vi "pp3_updateSideState.vi"(8 "error in (no error)":errorcluster, 9 "log queue in":refnum<queue>, 10 "Daq config In":T1={"Sound AO"="Dev6/ao0", "Shock intesity AO"="Dev6/ao1", "Code_LED DO"="Dev6/port1:2", "Switch DI"="Dev6/port1/line0", "Webcam"="cam9", "Sound AO task"="", "Sound card task"=0, "Shock intensity AO task"="", "Code_LED DO task"="", "Switch DI task"="", "AO <=> Sound card"=FALSE, "Sound card"=0, "sample rate"=100000.0, "Variable shock"=TRUE, "Webcam on"=FALSE, "Waveform memo"={"t0"=timestamp(0 s since 1904-01-01), "dt"=1.0, "Y"=[]}, "First time"=FALSE, "Tone trigger"="", "Master-9 DO"="Dev6/port0/line5:7"} {"sample rate" min=8000.0; "Sound card task" format="%.0x"}, 11 "State In":T4={"Curr  tr"=0, "Curr (ms)"=0, "Cum (ms)"=0, "Run loop diff"=0, "Tone countdown (ms)"=0, "Countdown (ms)"=0, "Curr State"=enum."0 NULL", "Prev State"=enum."1 Habituation", "Rw"=FALSE, "Sw"=FALSE, "Tone\nGate"=FALSE, "Punish"=FALSE, "Current DAQ DO Int"=0, "Current Loaded Trial"={"Trial Type Number"=1, "Trial Type"=enum."GO", "Trial Weight"=100, "Shock (mA)"=0.3, "Duration (ms)"=0.25, "Sound Type"=enum."04 FM Sweep", "Stim P1"=4000.0, "Stim P2"=0.0, "Stim P3"=0.0, "Stim P4"=2000.0, "DAQ Amplitude (V)"=0.25}, "Next Trial (for display purposes)"={"Trial Type Number"=1, "Trial Type"=enum."GO", "Trial Weight"=100, "Shock (mA)"=0.3, "Duration (ms)"=0.25, "Sound Type"=enum."04 FM Sweep", "Stim P1"=4000.0, "Stim P2"=0.0, "Stim P3"=0.0, "Stim P4"=2000.0, "DAQ Amplitude (V)"=0.25}, "Total trials memo"=0, "State start cum memo (ms)"=0, "Last dur jump time memo (ms)"=0, "Last dur shock time memo (ms)"=0, "Tone repeat memo (ms)"=0, "Webcam on"=FALSE, "Webcam recording"=FALSE, "State update flag"=FALSE, "Last loaded shock voltage"=0.0, "Vid upd"=enum."0"} {"Current DAQ DO Int" format="%016b"; "Next Trial (for display purposes)"."DAQ Amplitude (V)" min=0.0 max=5.0 format="%_4g"; "Next Trial (for display purposes)"."Shock (mA)" min=-1.0 max=5.0; "Next Trial (for display purposes)"."Trial Weight" step=1; "Next Trial (for display purposes)"."Duration (ms)" min=0.0 max=1.0; "Next Trial (for display purposes)"."Trial Type Number" min=1 max=256 step=1; "Current Loaded Trial"."DAQ Amplitude (V)" min=0.0 max=5.0 format="%_4g"; "Current Loaded Trial"."Shock (mA)" min=-1.0 max=5.0; "Current Loaded Trial"."Trial Weight" step=1; "Current Loaded Trial"."Duration (ms)" min=0.0 max=1.0; "Current Loaded Trial"."Trial Type Number" min=1 max=256 step=1}) -> (0 "error out":errorcluster, 1 "log queue out":refnum<queue>, 3 "State Out":T4={"Curr  tr"=0, "Curr (ms)"=0, "Cum (ms)"=0, "Run loop diff"=0, "Tone countdown (ms)"=0, "Countdown (ms)"=0, "Curr State"=enum."0 NULL", "Prev State"=enum."1 Habituation", "Rw"=FALSE, "Sw"=FALSE, "Tone\nGate"=FALSE, "Punish"=FALSE, "Current DAQ DO Int"=0, "Current Loaded Trial"={"Trial Type Number"=1, "Trial Type"=enum."GO", "Trial Weight"=100, "Shock (mA)"=0.3, "Duration (ms)"=0.25, "Sound Type"=enum."04 FM Sweep", "Stim P1"=4000.0, "Stim P2"=0.0, "Stim P3"=0.0, "Stim P4"=2000.0, "DAQ Amplitude (V)"=0.25}, "Next Trial (for display purposes)"={"Trial Type Number"=1, "Trial Type"=enum."GO", "Trial Weight"=100, "Shock (mA)"=0.3, "Duration (ms)"=0.25, "Sound Type"=enum."04 FM Sweep", "Stim P1"=4000.0, "Stim P2"=0.0, "Stim P3"=0.0, "Stim P4"=2000.0, "DAQ Amplitude (V)"=0.25}, "Total trials memo"=0, "State start cum memo (ms)"=0, "Last dur jump time memo (ms)"=0, "Last dur shock time memo (ms)"=0, "Tone repeat memo (ms)"=0, "Webcam on"=FALSE, "Webcam recording"=FALSE, "State update flag"=FALSE, "Last loaded shock voltage"=0.0, "Vid upd"=enum."0"} {"Current DAQ DO Int" format="%016b"; "Next Trial (for display purposes)"."DAQ Amplitude (V)" min=0.0 max=5.0 format="%_4g"; "Next Trial (for display purposes)"."Shock (mA)" min=-1.0 max=5.0; "Next Trial (for display purposes)"."Trial Weight" step=1; "Next Trial (for display purposes)"."Duration (ms)" min=0.0 max=1.0; "Next Trial (for display purposes)"."Trial Type Number" min=1 max=256 step=1; "Current Loaded Trial"."DAQ Amplitude (V)" min=0.0 max=5.0 format="%_4g"; "Current Loaded Trial"."Shock (mA)" min=-1.0 max=5.0; "Current Loaded Trial"."Trial Weight" step=1; "Current Loaded Trial"."Duration (ms)" min=0.0 max=1.0; "Current Loaded Trial"."Trial Type Number" min=1 max=256 step=1}, 4 "State timeout":bool, 5 "vid display":bool, 6 "Side change":bool)   [LabVIEW 2013]
uses:
  pp3_CTL_StateInfo.ctl
  pp3_CTL_State.ctl
  pp3_CTL_Trial.ctl
  pp3_CTL_TrialType.ctl
  labolabo2/waveforms/WFTypes.ctl
  pp3_CTL_DaqConfig.ctl
  <vilib>/userdefined/High Color/IMAQdx.ctl
  <vilib>/sound2/lvsound2.llb/Sound Output Task ID.ctl
  <vilib>/DAQmx/read.llb/DAQmx Read (Digital Bool 1Line 1Point).vi
  <vilib>/DAQmx/miscellaneous.llb/DAQmx Fill In Error Info.vi
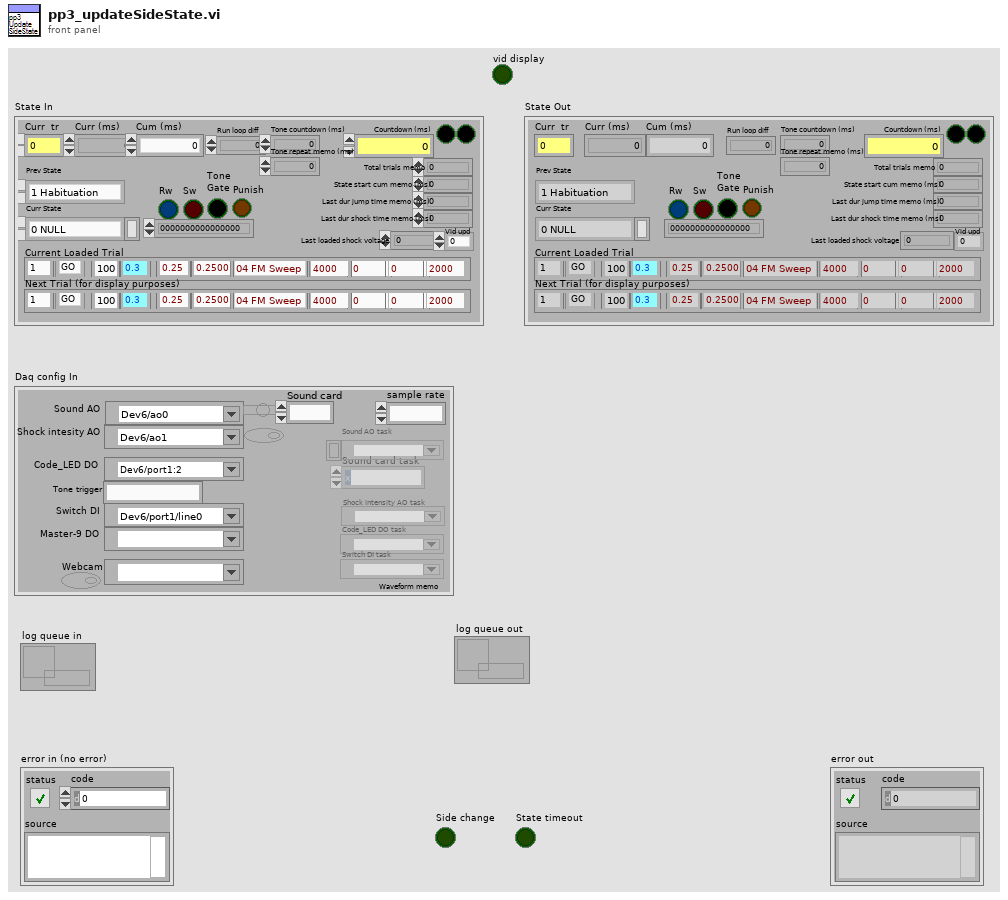
[diagram p1: front panel]
types:
  T1 = typedef "pp3_CTL_DaqConfig.ctl" = cluster{"Sound AO":tag, "Shock intesity AO":tag, "Code_LED DO":tag, "Switch DI":tag, "Webcam":T2, "Sound AO task":refnum<k21>, "Sound card task":T3, "Shock intensity AO task":refnum<k21>, "Code_LED DO task":refnum<k21>, "Switch DI task":refnum<k21>, "AO <=> Sound card":bool, "Sound card":u32, "sample rate":dbl, "Variable shock":bool, "Webcam on":bool, "Waveform memo":waveform(dbl), "First time":bool, "Tone trigger":string, "Master-9 DO":tag}
  T2 = typedef "IMAQdx.ctl" = refnum<k21>
  T3 = typedef "Sound Output Task ID.ctl" = u32
  T4 = typedef "pp3_CTL_StateInfo.ctl" = cluster{"Curr  tr":u16, "Curr (ms)":u32, "Cum (ms)":i64, "Run loop diff":i64, "Tone countdown (ms)":i64, "Countdown (ms)":i64, "Curr State":T5, "Prev State":T5, "Rw":bool, "Sw":bool, "Tone\nGate":bool, "Punish":bool, "Current DAQ DO Int":u16, "Current Loaded Trial":T6, "Next Trial (for display purposes)":T6, "Total trials memo":i64, "State start cum memo (ms)":i64, "Last dur jump time memo (ms)":i64, "Last dur shock time memo (ms)":i64, "Tone repeat memo (ms)":i64, "Webcam on":bool, "Webcam recording":bool, "State update flag":bool, "Last loaded shock voltage":dbl, "Vid upd":enum16{"0", "1", "2", "3", "4", "5", "6", "7", "8", "9"}}
  T5 = typedef "pp3_CTL_State.ctl" = enum8{"0 NULL", "1 Habituation", "2 (Load Trial)", "3 Stay Period", "4 Load Audio/Click Delay", "5 GO Trial", "6 GO Jumped", "7 GO Timeout", "8 NOGO Trial", "9 NOGO Jumped", "10 NOGO Timeout", "11 TEST Trial", "12 TEST Jumped", "13 TEST Timeout", "14 Intertrial Interval", "15 Done"}
  T6 = typedef "pp3_CTL_Trial.ctl" = cluster{"Trial Type Number":i16, "Trial Type":T7, "Trial Weight":u32, "Shock (mA)":dbl, "Duration (ms)":dbl, "Sound Type":T8, "Stim P1":dbl, "Stim P2":dbl, "Stim P3":dbl, "Stim P4":dbl, "DAQ Amplitude (V)":dbl}
  T7 = typedef "pp3_CTL_TrialType.ctl" = enum16{"OFF", "GO", "NOGO", "TEST"}
  T8 = typedef "WFTypes.ctl" = enum16{"00 NULL", "01 DC", "02 Noise", "03 Pure Tone", "04 FM Sweep"}
  T9 = enum16{"0", "1", "2", "3", "4", "5", "6", "7", "8", "9"}
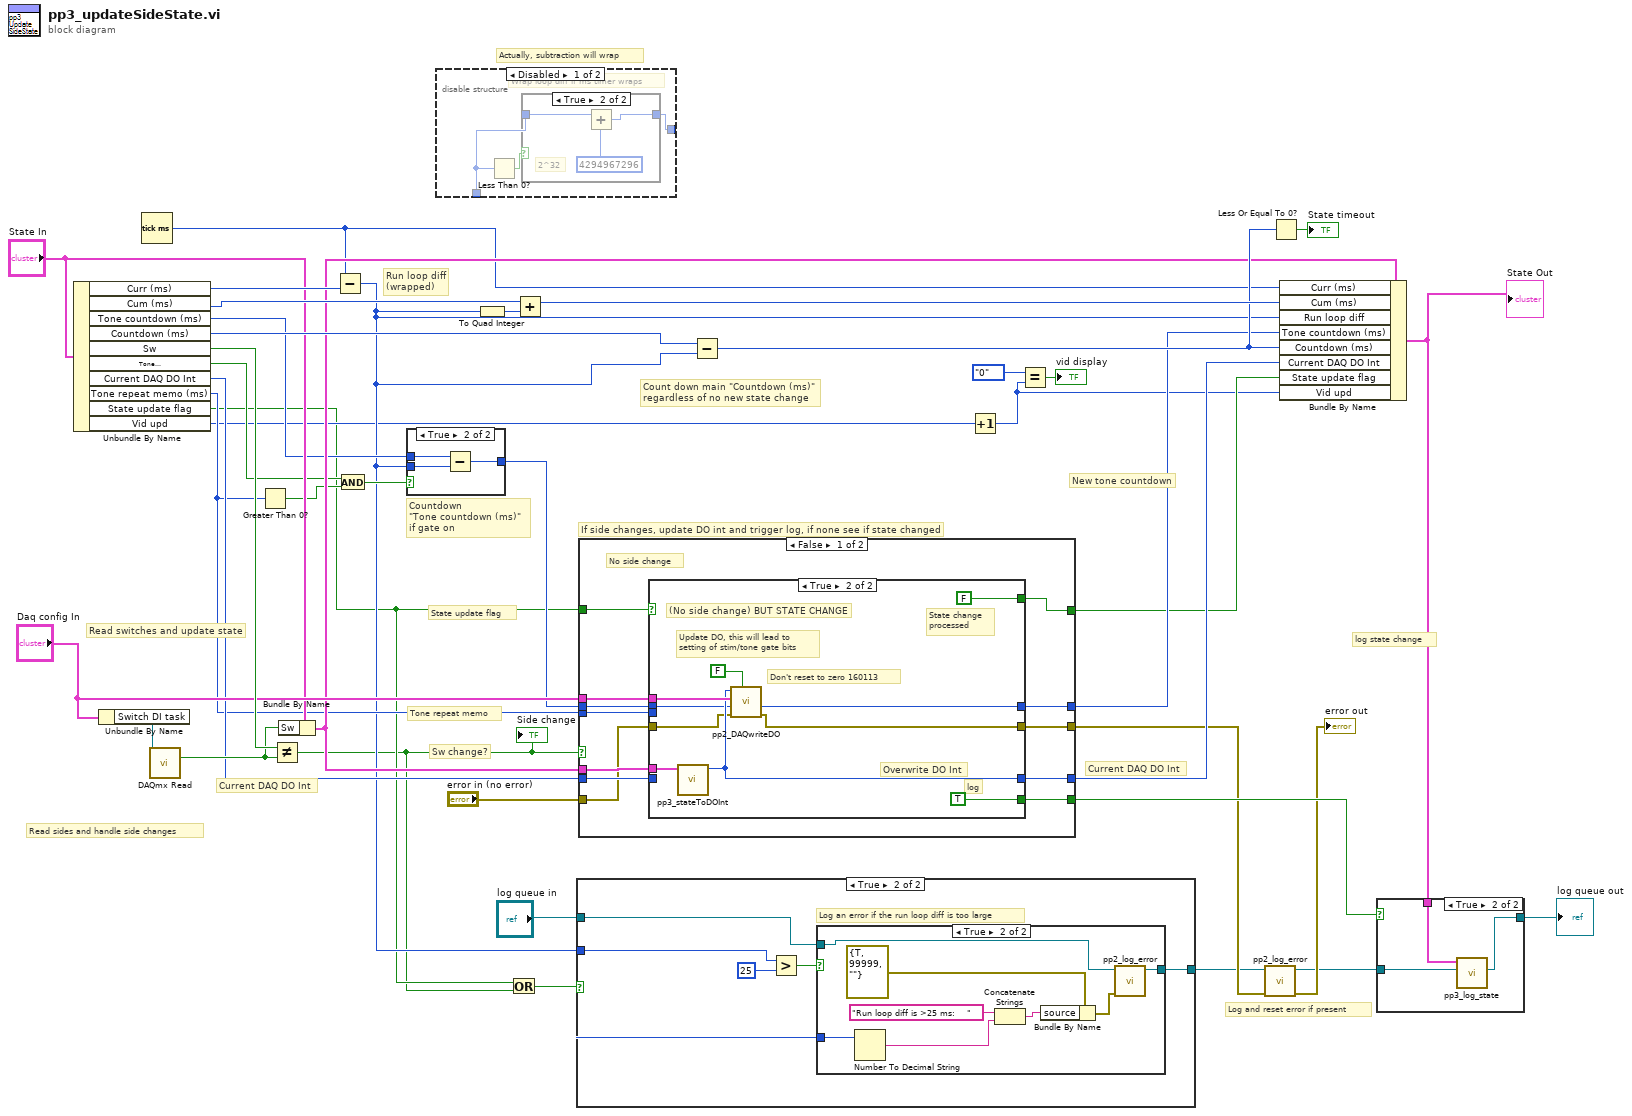
[diagram p0: block diagram]
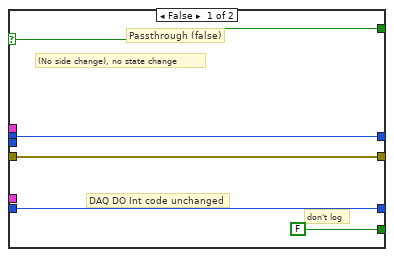
[diagram p8: hidden frame]
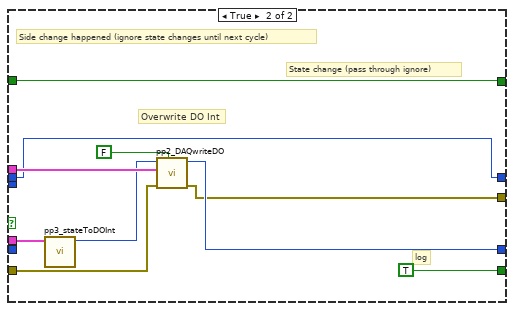
[diagram p9: hidden frame]
diagram:
  # "Actually, subtraction will wrap"
  # "Log and reset error if present"
  # "New tone countdown"
  # "Countdown \n\"Tone countdown (ms)\" \nif gate on"
  # "Read switches and update state"
  # "Tone repeat memo"
  # "Sw change?"
  # "Current DAQ DO Int"
  # "Current DAQ DO Int"
  # "Count down main \"Countdown (ms)\" \nregardless of no new state change"
  # "State update flag"
  # "Run loop diff\n(wrapped)"
  # "If side changes, update DO int and trigger log, if none see if state changed"
  # "Read sides and handle side changes"
  # "log state change"
  n1 = Unbundle By Name("State In") -> ("Curr (ms)"=w41:u32, "Cum (ms)"=w40:i64, "Tone countdown (ms)"=w25:i64, "Countdown (ms)"=w38:i64, "Sw"=w36:bool, "Tone\nGate"=w15:bool, "Current DAQ DO Int"=w17:u16, "Tone repeat memo (ms)"=w13:i64, "State update flag"=w2:bool, "Vid upd"=w7:T9)
  n2 = Unbundle By Name("Daq config In") -> ("Switch DI task"=w37:refnum<k21>)
  n3 = Tick Count (ms)() -> (millisecond timer value=w22:u32)
  n4 = call-poly <vilib>:"DAQmx Read.vi"("task/channels in"=w37) -> ("data"=w23:bool)  [unwired: 12 in, 2 out]
  n5 = Greater Than 0?(x=w13) -> (x > 0?=w14:bool)
  n6 = Not Equal?(x=w36, y=w23) -> (x != y?=w1:bool)
  "Side change" <- w1
  n7 = Bundle By Name(cluster="State In", "Sw"=w23) -> (w26:T4)
  n8 = Subtract(x=w22, y=w41) -> (x-y=w12:u32)
  n9 = And(x=w15, y=w14) -> (x .and. y?=w16:bool)
  n10 = case shown="True" w16 {
    tunnel: [w42 w43] -> w24
    tunnel: w25 -> [w42 w45]
    tunnel: w12 -> [_ w44]
    frame False {
      # "Passthrough if\ntone gate off"
    }
    frame True {
      n11 = Subtract(x=w45, y=w44) -> (x-y=w43:i64)
    }
  }
  n12 = disable-structure shown="Disabled" {
    disable-tunnel: [w47 _] -> _
    disable-tunnel: [w46 _] -> _
    frame Disabled {
      # "Wrap loop diff if ms timer wraps"
      n13 = Less Than 0?(x=w47) -> (x < 0?=w48:bool)
      n14 = case shown="True" w48 {
        tunnel: [w49 w51] -> w47
        tunnel: [w49 w52] -> w46
        frame False {
        }
        frame True {
          # "2^32"
          n15 = Add(x=w51, y=i64 4294967296) -> (x+y=w52:i64)
        }
      }
    }
    frame Enabled {
    }
  }
  n16 = To Quad Integer(1:w12) -> (0:w21:i64)
  n17 = Or(x=w2, y=w1) -> (x .or. y?=w3:bool)
  n18 = Add(x=w40, y=w21) -> (x+y=w39:i64)
  n19 = case shown="True" w3 {
    tunnel: w12 -> [_ w56]
    tunnel: "log queue in" -> [w53 w55]
    tunnel: [w53 w54] -> w10
    frame False {
    }
    frame True {
      # "Log an error if the run loop diff is too large"
      n20 = Greater?(x=w56, y=u32 25) -> (0:w57:bool)
      n21 = case shown="True" w57 {
        tunnel: w56 -> [_ w66]
        tunnel: w55 -> [w59 w61]
        tunnel: [w59 w60] -> w54
        frame False {
        }
        frame True {
          n22 = Number To Decimal String(number=w66) -> (decimal integer string=w63:string)  [unwired: 1 in]
          n23 = Concatenate Strings("Run loop diff is >25 ms:    " ("string"), w63) -> (w65:string)
          n24 = Bundle By Name(cluster=errorcluster {"status"=TRUE, "code"=99999, "source"=""} ("error in (no error)"), "source"=w65) -> (w62:errorcluster)
          n25 = call "pp2_log_error.vi"("error in (no error)"=w62, "queue in"=w61) -> ("queue out"=w60:refnum<queue>)  [unwired: 6 in, 1 out]
        }
      }
    }
  }
  n26 = case shown="False" w1 {
    tunnel: "Daq config In" -> [w73 w101]
    tunnel: [w78 w100] -> w27
    tunnel: w17 -> [w79 _]
    tunnel: "error in (no error)" -> [w72 w99]
    tunnel: [w76 w98] -> w19
    tunnel: [w77 TRUE] -> w31
    tunnel: w13 -> [w71 _]
    tunnel: w2 -> [w75 w95]
    tunnel: w26 -> [w74 w97]
    tunnel: [w70 w96] -> w29
    tunnel: w24 -> [w69 w96]
    tunnel: [w68 w95] -> w20
    frame False {
      # "No side change"
      n27 = case shown="True" w75 {
        selector: w75 -> [w81 _]
        tunnel: w79 -> [w80 _]
        tunnel: [w80 w92] -> w78
        tunnel: w73 -> [_ w93]
        tunnel: [FALSE TRUE] -> w77
        tunnel: w72 -> [w82 w90]
        tunnel: [w82 w89] -> w76
        tunnel: w74 -> [_ w88]
        tunnel: w69 -> [w83 w87]
        tunnel: w71 -> [_ _]
        tunnel: [w83 w87] -> w70
        tunnel: [w81 FALSE] -> w68
        frame False {
          # "Passthrough (false)"
          # "don't log"
          # "DAQ DO Int code unchanged"
          # "(No side change), no state change"
        }
        frame True {
          # "Don't reset to zero 160113"
          # "State change\nprocessed"
          # "log"
          # "Overwrite DO Int"
          # "Update DO, this will lead to\nsetting of stim/tone gate bits"
          # "(No side change) BUT STATE CHANGE"
          n28 = call "pp3_stateToDOInt.vi"("State In"=w88) -> ("DAQ Output Int"=w92:u16)  [unwired: 10 in]
          n29 = call "pp2_DAQwriteDO.vi"("Reset to zero"=FALSE, "error in (no error)"=w90, "Daq config"=w93, "DAQ Digital In"=w92) -> ("error out"=w89:errorcluster)  [unwired: 7 in]
        }
      }
    }
    frame True {
      # "State change (pass through ignore)"
      # "log"
      # "Side change happened (ignore state changes until next cycle)"
      # "Overwrite DO Int"
      n30 = call "pp3_stateToDOInt.vi"("State In"=w97) -> ("DAQ Output Int"=w100:u16)  [unwired: 10 in]
      n31 = call "pp2_DAQwriteDO.vi"("Reset to zero"=FALSE, "error in (no error)"=w99, "Daq config"=w101, "DAQ Digital In"=w100) -> ("error out"=w98:errorcluster)  [unwired: 7 in]
    }
  }
  n32 = Subtract(x=w38, y=w12) -> (x-y=w35:i64)
  n33 = Increment(x=w7) -> (x+1=w6:T9)
  n34 = Equal?(x=T9."0", y=w6) -> (x = y?=→"vid display":bool)
  n35 = call "pp2_log_error.vi"("error in (no error)"=w19, "queue in"=w10) -> ("error out"=→"error out":errorcluster, "queue out"=w9:refnum<queue>)  [unwired: 6 in]
  n36 = Less Or Equal To 0?(x=w35) -> (x <= 0?=→"State timeout":bool)
  n37 = Bundle By Name(cluster=w26, "Curr (ms)"=w22, "Cum (ms)"=w39, "Run loop diff"=w12, "Tone countdown (ms)"=w29, "Countdown (ms)"=w35, "Current DAQ DO Int"=w27, "State update flag"=w20, "Vid upd"=w6) -> (w30:T4)
  "State Out" <- w30
  n38 = case shown="True" w31 {
    tunnel: w30 -> [_ w106]
    tunnel: w9 -> [w103 w105]
    tunnel: [w103 w104] -> w8
    frame False {
    }
    frame True {
      n39 = call "pp3_log_state.vi"("queue in"=w105, "State In"=w106) -> ("queue out"=w104:refnum<queue>)  [unwired: 9 in]
    }
  }
  "log queue out" <- w8
